vi "Save Window.vi"(0 "LV MDI in":refnum<class "LV MDI.lvclass">, 5 "ChildHwnd[]":u32[](array[numeric]), 11 "error in (no error)":errorcluster) -> (4 "LV MDI out":refnum<class "LV MDI.lvclass">, 6 "Displayed Doc[]":string[](array[string]), 8 "Position[]":T1[](array[typedef]), 15 "error out":errorcluster)   [LabVIEW 2016, in "LV MDI.lvclass"]
uses:
  LV MDI.lvclass
  TypeDefs/Set Position.ctl
  TypeDefs/Offset Rect.ctl
  LV MDI.lvclass/LV MDI.ctl
  Document/Document.lvclass/Document.ctl
  user32.dll
  Document/Document.lvclass
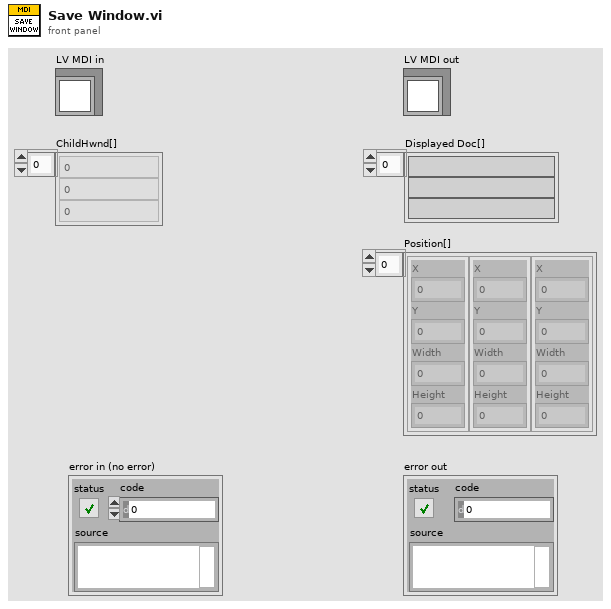
[diagram p1: front panel]
types:
  T1 = typedef "LV MDI.lvclass/Set Position.ctl" = cluster{"X":i32, "Y":i32, "Width":i32, "Height":i32}
  T2 = typedef "LV MDI.lvclass/Offset Rect.ctl" = cluster{"Left":i32, "Top":i32, "Right":i32, "Bottom":i32}
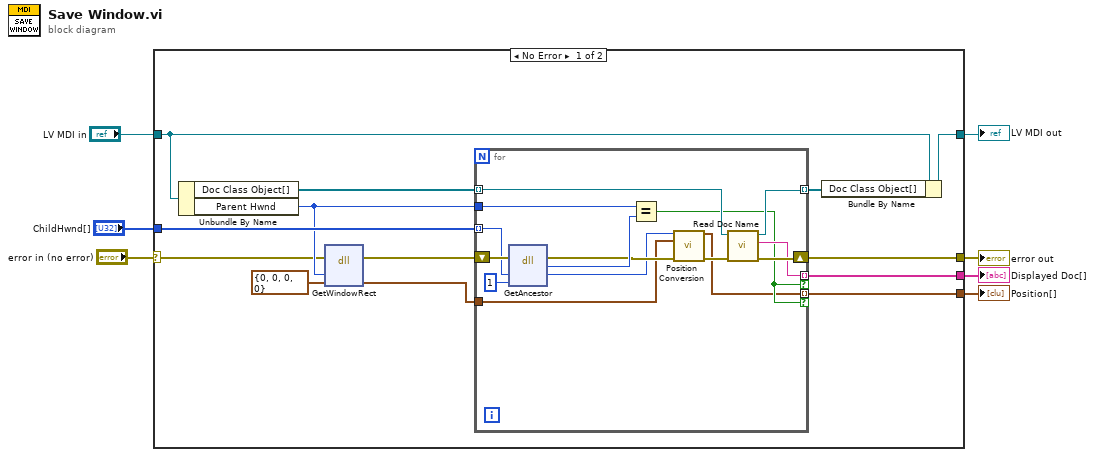
[diagram p0: block diagram]
diagram:
  n1 = case shown="No Error" "error in (no error)" {
    selector: "error in (no error)" -> [w11 w37]
    tunnel: "ChildHwnd[]" -> [w20 _]
    tunnel: [w19 w37] -> w5
    tunnel: "LV MDI in" -> [w17 w36]
    tunnel: [w16 w36] -> w3
    tunnel: [w14 _] -> w2
    tunnel: [w13 _] -> w1
    frame No Error {
      n2 = Unbundle By Name(w17) -> ("Doc Class Object[]"=w18:refnum<class "Document.lvclass">[], "Parent Hwnd"=w12:i32)
      n3 = dll-call lib="user32.dll" fn="GetWindowRect"(error in=w11, "Hwnd"=w12, "lpRect"=T2 {"Left"=0, "Top"=0, "Right"=0, "Bottom"=0} ("Offset Rect")) -> (error out=w10:errorcluster, "lpRect"=w8:T2)  [unwired: 4 in, 1 out]
      n4 = for {
        shift-right: [w29] -> w19
        shift-left: w10 -> [w35]
        tunnel: w20 -> [w34] mode=indexing
        tunnel: w12 -> [w32]
        tunnel: [w26] -> w14 mode=indexing if=w23
        tunnel: w18 -> [w28] mode=indexing
        tunnel: [w27] -> w15 mode=indexing
        tunnel: [w22] -> w13 mode=indexing if=w23
        tunnel: w8 -> [w21]
        n5 = dll-call lib="user32.dll" fn="GetAncestor"(error in=w35, "Hwnd"=w34, "gaflags"=1) -> (error out=w30:errorcluster, "Parent"=w31:i32, "Hwnd"=w24:u32)  [unwired: 3 in, 1 out]
        n6 = Equal?(x=w32, y=w31) -> (x = y?=w23:bool)
        n7 = call "Position Conversion.vi"("Child Hwnd"=w24, "Parent Position"=w21, "error in (no error)"=w30) -> ("Child Position"=w22:T1, "error out"=w25:errorcluster)  [unwired: 11 in]
        n8 = call "Read Doc Name.vi"("error in (no error)"=w25, "Document in"=w28) -> ("error out"=w29:errorcluster, "Doc Name"=w26:string, "Document out"=w27:refnum<class "Document.lvclass">)  [unwired: 7 in]
      }
      n9 = Bundle By Name(cluster=w17, "Doc Class Object[]"=w15) -> (w16:refnum<class "LV MDI.lvclass">)
    }
    frame Error {
    }
  }
  "error out" <- w5
  "LV MDI out" <- w3
  "Displayed Doc[]" <- w2
  "Position[]" <- w1
